vi "send rel move to stage.vi"(8 "error in (no error)":errorcluster, 9 "relative focus step":dbl[unit], 10 "relative z step":dbl[unit], 11 "Autofocus in":refnum<class "Autofocus.lvclass">) -> (0 "error out":errorcluster, 3 "Autofocus out":refnum<class "Autofocus.lvclass">)   [LabVIEW 2012, in "Autofocus.lvclass"]
uses:
  Autofocus.lvclass
  <vilib>/Distrio/Murmex/GenericMessage/GenericMessage.lvclass
  <vilib>/Distrio/Murmex/StartMessage/StartMessage.lvclass
  Autofocus.lvclass/Autofocus.ctl
  <vilib>/Distrio/Murmex/Message/Message.lvclass
  <vilib>/Distrio/Murmex/Murmex/Murmex.lvclass
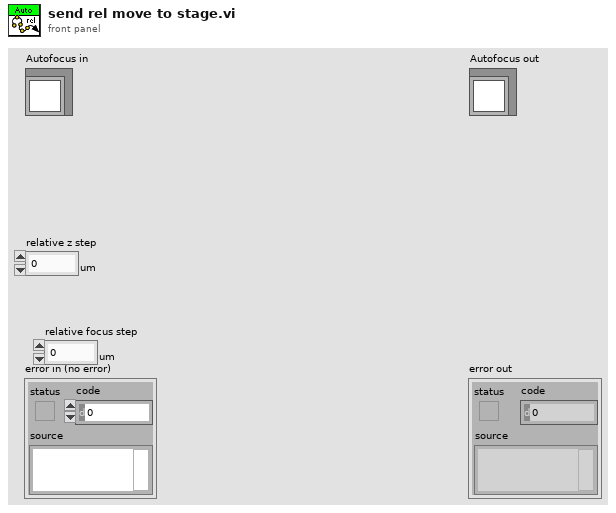
[diagram p1: front panel]
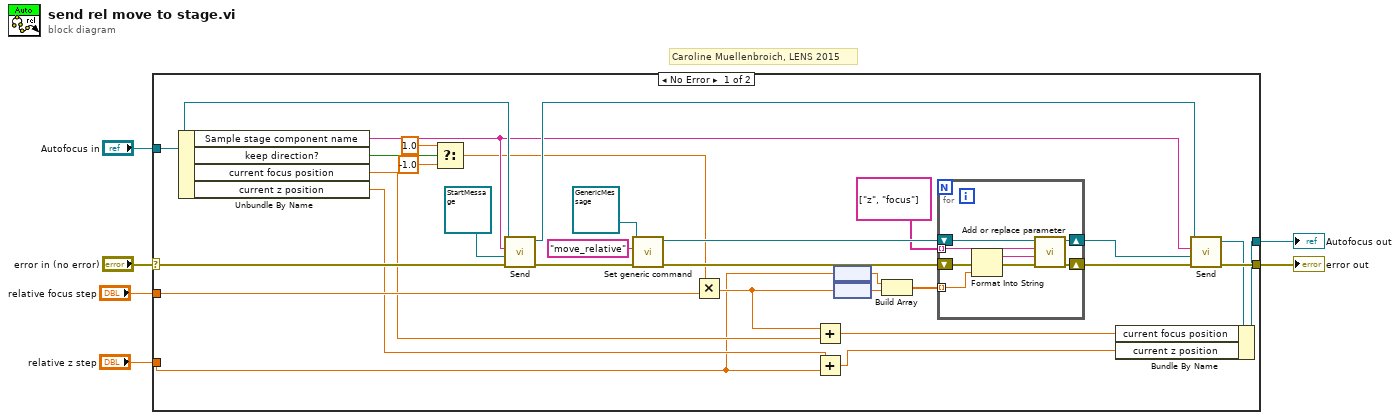
[diagram p0: block diagram]
diagram:
  # "Caroline Muellenbroich, LENS 2015"
  n1 = case shown="No Error" "error in (no error)" {
    selector: "error in (no error)" -> [w24 w46]
    tunnel: [w34 w46] -> w5
    tunnel: [w28 w45] -> w3
    tunnel: "Autofocus in" -> [w22 w45]
    tunnel: "relative z step" -> [w9 _]
    tunnel: "relative focus step" -> [w16 _]
    frame No Error {
      n2 = Unbundle By Name(w22) -> ("Sample stage component name"=w19:string, "keep direction?"=w27:bool, "current focus position"=w15:dbl[unit], "current z position"=w11:dbl[unit])
      n3 = Select(t=1.0, s=w27, f=-1.0) -> (s? t:f=w17:dbl)
      n4 = call <vilib>:"Send.vi"("error in (no error)"=w24, "Message"=refnum<class "StartMessage.lvclass"> refnum ("Message in"), "recipient"=w19, "Murmex in"=w22) -> ("error out"=w23:errorcluster, "Murmex out"=w21:refnum<class "Autofocus.lvclass">)  [unwired: 6 in]
      n5 = call <vilib>:"Set generic command.vi"("error in (no error)"=w23, "generic command"="move_relative" ("command string"), "GenericMessage in"=refnum<class "GenericMessage.lvclass"> refnum ("Murmex.lvlib:GenericMessage")) -> ("error out"=w31:errorcluster, "GenericMessage out"=w30:refnum<class "GenericMessage.lvclass">)  [unwired: 7 in]
      n6 = Multiply(x=w17, y=w16) -> (x*y=w13:dbl[unit])
      n7 = Add(x=w13, y=w15) -> (x+y=w8:dbl[unit])
      n8 = Add(x=w11, y=w9) -> (x+y=w7:dbl[unit])
      n9 = node(w9) -> (w10:dbl)
      n10 = node(w13) -> (w14:dbl)
      n11 = Build Array(w10, w14) -> (w12:dbl[])
      n12 = for {
        tunnel: string[] ["z", "focus"] -> [w42] mode=indexing
        shift-right: [w43] -> w35
        shift-left: w31 -> [w39]
        shift-right: [w44] -> w36
        shift-left: w30 -> [w38]
        tunnel: w12 -> [w37] mode=indexing
        n13 = Format Into String(error in=w39, w37) -> (resulting string=w41:string, error out=w40:errorcluster)  [unwired: 2 in]
        n14 = call <vilib>:"Add or replace parameter.vi"("error in (no error)"=w40, "value"=w41, "name"=w42, "Message in"=w38) -> ("error out"=w43:errorcluster, "Message out"=w44:refnum<class "GenericMessage.lvclass">)  [unwired: 6 in]
      }
      n15 = call <vilib>:"Send.vi"("error in (no error)"=w35, "Message"=w36, "recipient"=w19, "Murmex in"=w21) -> ("error out"=w34:errorcluster, "Murmex out"=w29:refnum<class "Autofocus.lvclass">)  [unwired: 6 in]
      n16 = Bundle By Name(cluster=w29, "current focus position"=w8, "current z position"=w7) -> (w28:refnum<class "Autofocus.lvclass">)
    }
    frame Error {
    }
  }
  "error out" <- w5
  "Autofocus out" <- w3
